vi "SimpleConnectAndPublish.vi"() -> ()   [LabVIEW 2018, in "AWS_IoT.lvlib"]
uses:
  AWS_IoT.lvlib
  MQTT/Controls/QoS.ctl
  MQTT/Controls/Retain_Flag.ctl
  MQTT/Controls/DUP_Flag.ctl
  Controls/certs.ctl
  MQTT/Controls/Connection_Return_Codes.ctl
  MQTT/Controls/ConnectMeta.ctl
  MQTT/Controls/Will_Info.ctl
  MQTT/Controls/Connect_Flags.ctl
panel:
  out "length":i32
  in  "Publish?":bool=TRUE
  in  "millisecond multiple":u32=1000
  in  "Will Info":T1={"Will message"="Last Will", "Will Topic"="Will Topic"}
  in  "Connect Meta":T2={"Retain"=TRUE, "DUP"=FALSE, "Keep Alive (sec)"=60, "QoS"=enum."At most once"}
  out "Connection Status":T6=enum."Connection refused: not authorized"
  in  "cert path":T7={"client cert file"=path "", "client key file"=path ""}
  in  "Publish Meta":cluster{"QoS":T5, "Retain":T3, "DUP":T4}
  in  "Topic":string="testtopic/LVMQTT"
  in  "error in (no error)":errorcluster
  in  "Client ID":string="LabVIEW_MQTT_Client"
  out "error out":errorcluster
  in  "Message to be published":string="LabVIEW says it's "
  in  "MQTT Broker":cluster{"address (IP)":string, "port":u16}={"address (IP)"="a28e3t2sj3ekjh.iot.us-west-2.amazonaws.com", "port"=8883}
  in  "Message ID":u16=20
  in  "Stop Publishing":bool
  out "Message published":string
  out "Message ID (acknowledged)":u16=10
  out "Acknowledged":bool
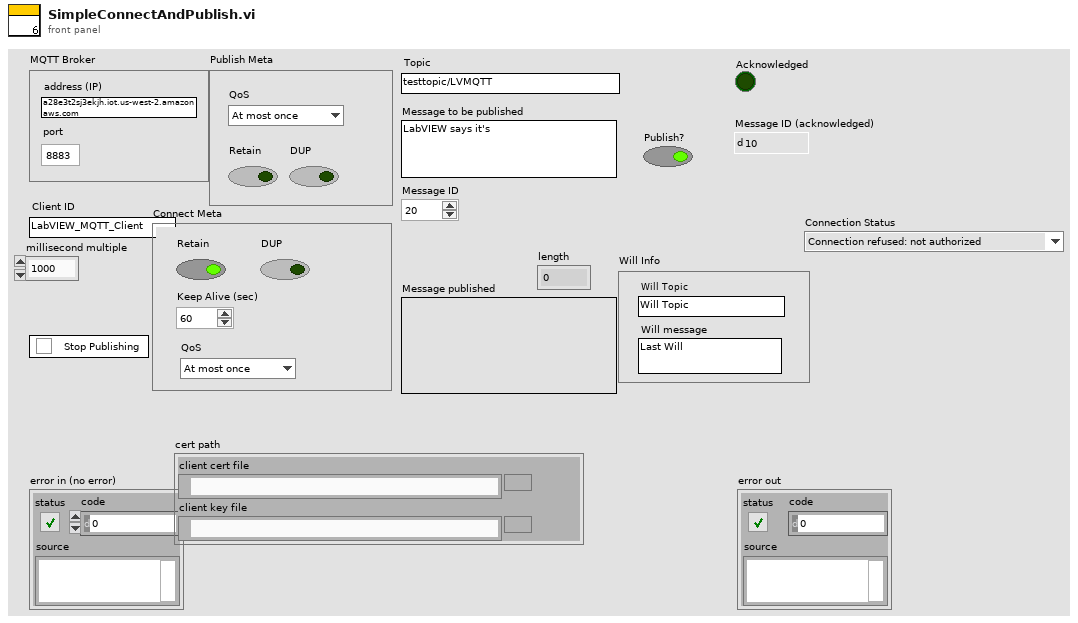
[diagram p1: front panel]
types:
  T1 = typedef "AWS_IoT.lvlib/Will_Info.ctl" = cluster{"Will message":string, "Will Topic":string}
  T2 = typedef "AWS_IoT.lvlib/ConnectMeta.ctl" = cluster{"Retain":T3, "DUP":T4, "Keep Alive (sec)":u16, "QoS":T5}
  T3 = typedef "AWS_IoT.lvlib/Retain_Flag.ctl" = bool
  T4 = typedef "AWS_IoT.lvlib/DUP_Flag.ctl" = bool
  T5 = typedef "AWS_IoT.lvlib/QoS.ctl" = enum8{"At most once", "At least once", "Exactly once", "Reserved"}
  T6 = typedef "AWS_IoT.lvlib/Connection_Return_Codes.ctl" = enum16{"Connection accepted", "Connection refused: unacceptable protocol version", "Connection refused: identifier rejected", "Connection refused: Server unavailable", "Connection refused: bad user name or password", "Connection refused: not authorized"}
  T7 = typedef "AWS_IoT.lvlib/certs.ctl" = cluster{"client cert file":path, "client key file":path}
  T8 = typedef "AWS_IoT.lvlib/Connect_Flags.ctl" = cluster{"user name":bool, "password":bool, "will retain":bool, "will flag":bool, "clean session":bool, "reserved":bool, "will QoS":T5}
  T9 = typedef "AWS_IoT.lvlib/SSL_Connection.ctl" = cluster{"connection ID":refnum<k5>, "TLS":cluster{"CXT ptr":i32, "SSL ptr":i32, "Socket ptr":i32}, "NIssleay library path":path, "server url":string}
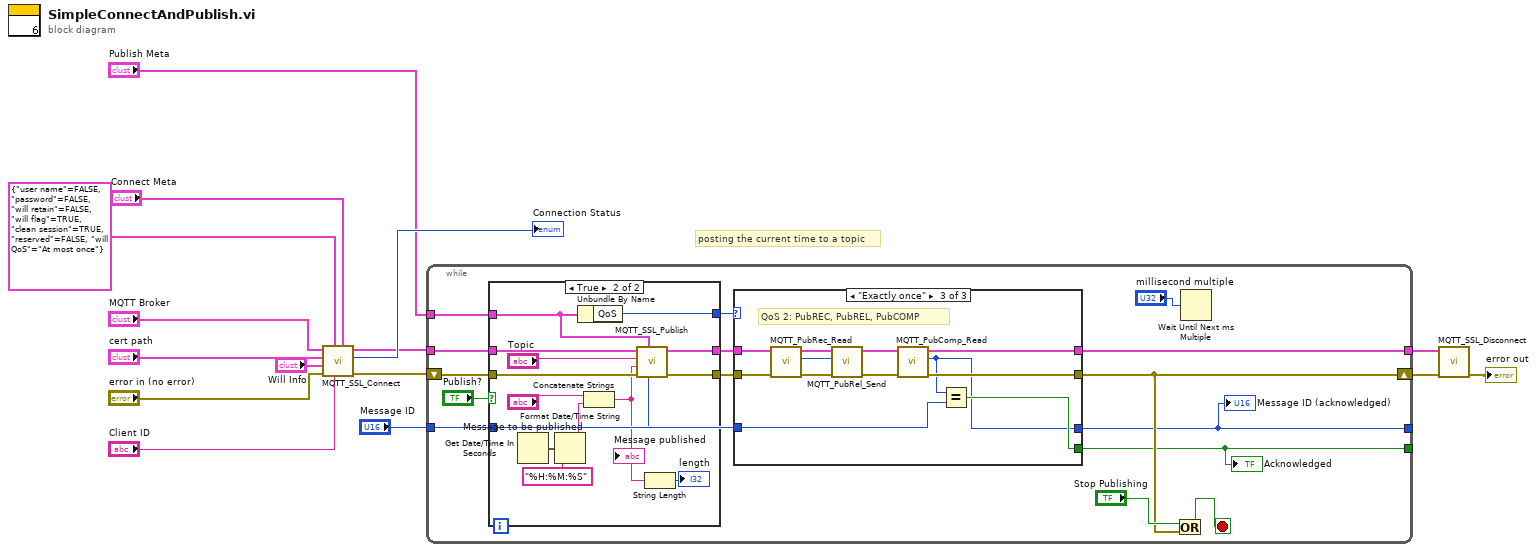
[diagram p0: block diagram]
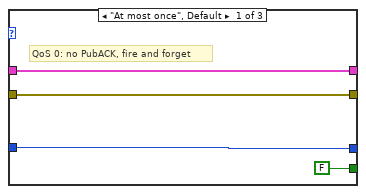
[diagram p3: hidden frame]
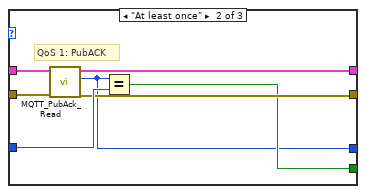
[diagram p4: hidden frame]
diagram:
  # "posting the current time to a topic"
  n1 = call "MQTT_SSL_Connect.vi"("Connect Meta"="Connect Meta", "Client ID"="Client ID", "Connect Flags"=T8 {"user name"=FALSE, "password"=FALSE, "will retain"=FALSE, "will flag"=TRUE, "clean session"=TRUE, "reserved"=FALSE, "will QoS"=enum."At most once"}, "error in (no error)"="error in (no error)", "Will Info"="Will Info", "cert path"="cert path", "MQTT Broker"="MQTT Broker") -> ("error out"=w15:errorcluster, "Connection Status"=→"Connection Status":T6, "SSL_Connection"=w13:T9)  [unwired: 2 in]
  n2 = while {
    tunnel: w13 -> [w17]
    tunnel: "Publish Meta" -> [w29]
    tunnel: [w25] -> w10
    tunnel: "Message ID" -> [w24]
    tunnel: [w19] -> _
    tunnel: [w18] -> _
    shift-right: [w21] -> w9
    shift-left: w15 -> [w30]
    stop <- w22 stop-if-true
    n3 = case shown="True" "Publish?" {
      tunnel: w30 -> [w31 w46]
      tunnel: w29 -> [_ w45]
      tunnel: [_ w44] -> w28
      tunnel: [w31 w43] -> w27
      tunnel: [w32 w42] -> w26
      tunnel: w24 -> [_ w41]
      tunnel: w17 -> [w32 w37]
      frame False {
      }
      frame True {
        n4 = Get Date/Time In Seconds() -> (seconds since 1Jan1904=w40:timestamp)
        n5 = Format Date/Time String(time format string (%c)="%H:%M:%S", seconds (now)=w40) -> (date/time string=w38:string)  [unwired: 1 in]
        n6 = Unbundle By Name(w45) -> ("QoS"=w44:T5)
        n7 = Concatenate Strings("Message to be published", w38) -> (w34:string)
        "Message published" <- w34
        n8 = call "MQTT_SSL_Publish.vi"("Message ID"=w41, "Publish Meta"=w45, "error in (no error)"=w46, "Message to be published"=w34, "Topic"="Topic", "SSL_Connection"=w37) -> ("error out"=w43:errorcluster, "SSL_Connection"=w42:T9)  [unwired: 4 in]
        n9 = String Length(string=w34) -> (length=→"length":i32)
      }
    }
    n10 = case shown="\"Exactly once\"" w28 {
      tunnel: w27 -> [w49 w56 w68]
      tunnel: w26 -> [w50 w57 w69]
      tunnel: [w49 w54 w61] -> w21
      tunnel: [w50 w53 w62] -> w25
      tunnel: w24 -> [w47 w55 w67]
      tunnel: [FALSE w52 w63] -> w19
      tunnel: [w47 w51 w60] -> w18
      frame "At most once", Default {
        # "QoS 0: no PubACK, fire and forget"
      }
      frame "At least once" {
        # "QoS 1: PubACK"
        n11 = call "MQTT_PubAck_Read.vi"("error in (no error)"=w56, "SSL_Connection"=w57) -> ("error out"=w54:errorcluster, "Message ID"=w51:u16, "SSL_Connection"=w53:T9)  [unwired: 7 in]
        n12 = Equal?(x=w51, y=w55) -> (x = y?=w52:bool)
      }
      frame "Exactly once" {
        # "QoS 2: PubREC, PubREL, PubCOMP"
        n13 = call "MQTT_PubRec_Read.vi"("error in (no error)"=w68, "SSL_Connection"=w69) -> ("error out"=w66:errorcluster, "Message ID"=w64:u16, "SSL_Connection"=w65:T9)  [unwired: 7 in]
        n14 = call "MQTT_PubRel_Send.vi"("error in (no error)"=w66, "Message ID"=w64, "SSL_Connection"=w65) -> ("error out"=w58:errorcluster, "SSL_Connection"=w59:T9)  [unwired: 6 in, 1 out]
        n15 = call "MQTT_PubComp_Read.vi"("error in (no error)"=w58, "SSL_Connection"=w59) -> ("error out"=w61:errorcluster, "Message ID"=w60:u16, "SSL_Connection"=w62:T9)  [unwired: 7 in]
        n16 = Equal?(x=w60, y=w67) -> (x = y?=w63:bool)
      }
    }
    "Message ID (acknowledged)" <- w18
    "Acknowledged" <- w19
    n17 = Or(x="Stop Publishing", y=w21) -> (x .or. y?=w22:bool)
    n18 = Wait Until Next ms Multiple(millisecond multiple="millisecond multiple") -> ()  [unwired: 1 out]
  }
  n19 = call "MQTT_SSL_Disconnect.vi"("error in (no error)"=w9, "SSL_Connection"=w10) -> ("error out"=→"error out":errorcluster)  [unwired: 9 in]
